vi "PRL UTIL Convert Command for Display.vi"(11 "Command In":string) -> (3 "Command Out":string)   [LabVIEW 2018, in "S3DK.lvlib" / "PMU Recorder Light.lvlib"]
doc: "Reformats the command string to be appropriate for display."
uses:
  .S3DK - Copy/PMU Recorder Light/PMU Recorder Light.lvlib
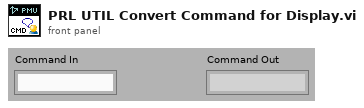
[diagram p1: front panel]
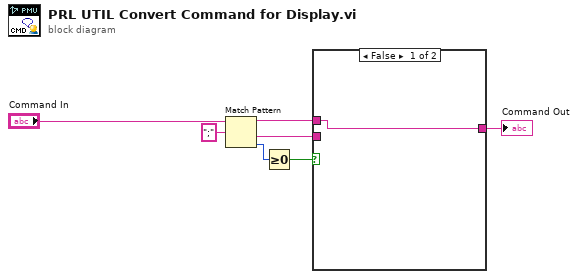
[diagram p0: block diagram]
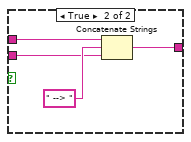
[diagram p2: hidden frame]
diagram:
  n1 = Match Pattern(string="Command In", regular expression=";") -> (before substring=w3:string, after substring=w2:string, offset past match=w5:i32)  [unwired: 1 in, 1 out]
  n2 = Greater Or Equal To 0?(x=w5) -> (x >= 0?=w4:bool)
  n3 = case shown="False" w4 {
    tunnel: w3 -> [w8 w11]
    tunnel: w2 -> [_ w10]
    tunnel: [w8 w9] -> w1
    frame False {
    }
    frame True {
      n4 = Concatenate Strings(w11, " --> ", w10) -> (w9:string)
    }
  }
  "Command Out" <- w1
